vi "ff_retag_blocks.vi"(8 "error in (no error)":errorcluster) -> (0 "error out":errorcluster)   [LabVIEW 2016]
uses:
  Typedef/comm_variable_definition.ctl
  Typedef/Comm_mode_type_combo.ctl
  Typedef/Comm_mode_and_address_type.ctl
panel:
  in  "Comm variable definitions":T1[](array[typedef]) {"Cluster"."Mode" items=["None", "MODBUS", "HART", "Profibus DP", "Profibus PA", "Fieldbus", "DeviceNET"]}
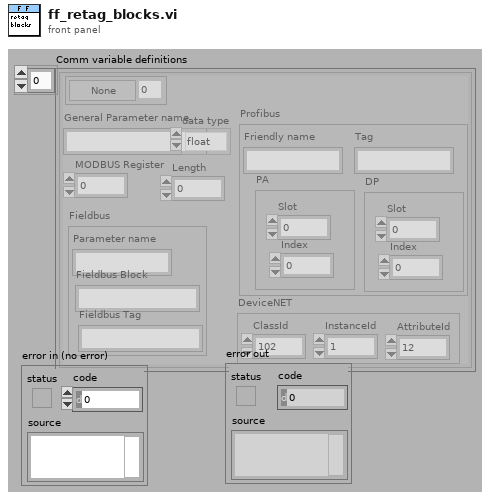
[diagram p1: front panel]
types:
  T1 = typedef "comm_variable_definition.ctl" = cluster{"General Parameter name":string, "MODBUS Register":i32, "Profibus":cluster{"Friendly name":string, "PA":cluster{"Slot":i32, "Index":i32}, "DP":cluster{"Slot":i32, "Index":i32}, "Tag":string}, "Fieldbus":cluster{"Parameter name":string, "Fieldbus Block":string, "Fieldbus Tag":string}, "data type":enum16{"float", "UINT", "UINT32", "STRING"}, "DeviceNET":cluster{"ClassId":u16, "InstanceId":u16, "AttributeId":u8}, "Cluster":T2, "Length":i32}
  T2 = typedef "Comm_mode_and_address_type.ctl" = cluster{"address":i32, "Mode":T3}
  T3 = typedef "Comm_mode_type_combo.ctl" = u16
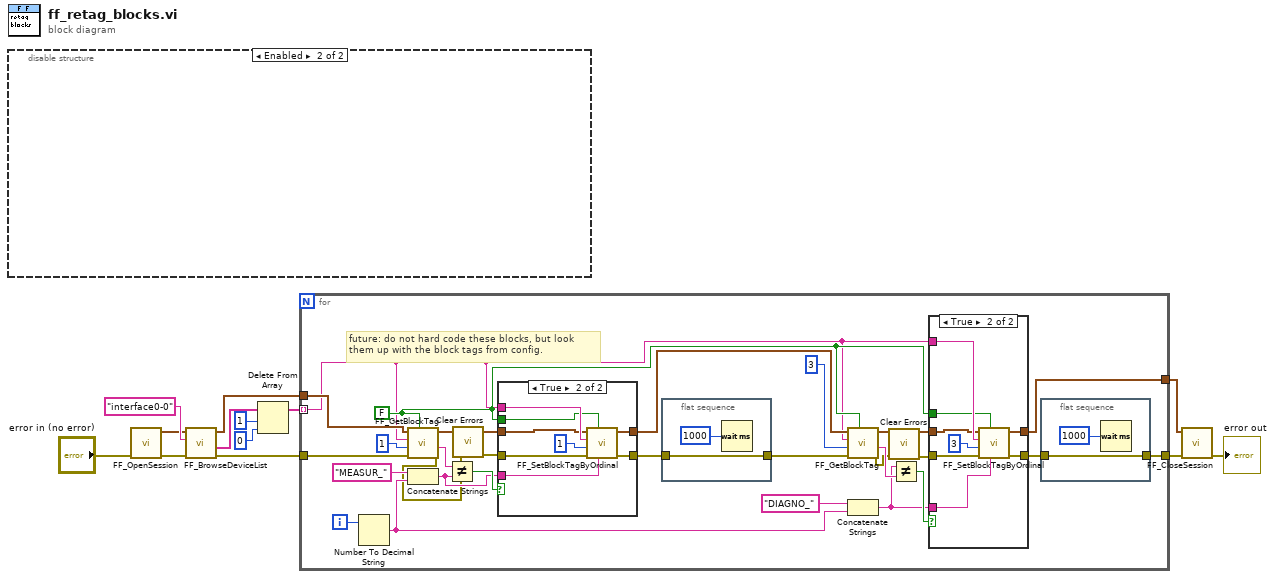
[diagram p0: block diagram]
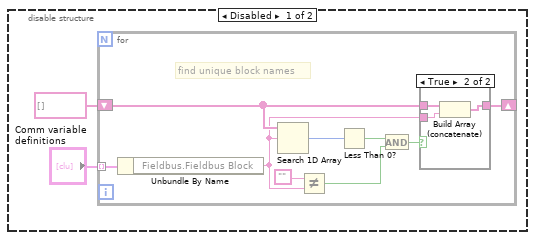
[diagram p2: hidden frame]
diagram:
  n1 = disable-structure shown="Enabled" {
    frame Disabled {
      n2 = for {
        tunnel: "Comm variable definitions" -> [w24] mode=indexing
        shift-right: [w21] -> _
        shift-left: string[] [] -> [w20]
        # "find unique block names"
        n3 = Unbundle By Name(w24) -> ("Fieldbus.Fieldbus Block"=w16:string)
        n4 = Search 1D Array(1D array=w20, element=w16) -> (index of element=w19:i32)  [unwired: 1 in]
        n5 = Not Equal?(x="", y=w16) -> (x != y?=w22:bool)
        n6 = Less Than 0?(x=w19) -> (x < 0?=w17:bool)
        n7 = And(x=w17, y=w22) -> (x .and. y?=w18:bool)
        n8 = case shown="True" w18 {
          tunnel: w16 -> [_ w28]
          tunnel: [w25 w27] -> w21
          tunnel: w20 -> [w25 w26]
          frame False {
          }
          frame True {
            n9 = Build Array (concatenate)(w26, w28) -> (w27:string[])
          }
        }
      }
    }
    frame Enabled {
    }
  }
  n10 = call "FF_OpenSession.vi"("error in (no error)"="error in (no error)") -> ("error out"=w9:errorcluster, "refnum out"=w8:cluster{"Handle1":u32, "Handle2":u32})  [unwired: 9 in]
  n11 = call "FF_BrowseDeviceList.vi"("error in (no error)"=w9, "link name"="interface0-0", "refnum in"=w8) -> ("error out"=w5:errorcluster, "deviceID list"=w13:string[], "refnum out"=w6:cluster{"Handle1":u32, "Handle2":u32})  [unwired: 4 in, 2 out]
  n12 = Delete From Array(array=w13, length=1, index=0) -> (array with subset deleted=w7:string[])  [unwired: 1 out]
  n13 = for {
    tunnel: w7 -> [w39] mode=indexing
    tunnel: [w33] -> w3
    tunnel: w6 -> [w52]
    tunnel: w5 -> [w47]
    tunnel: [w37] -> w4
    i -> [w55]
    w40 = FALSE ("Is pdTag")
    # "future: do not hard code these blocks, but look \nthem up with the block tags from config."
    n14 = Number To Decimal String(number=w55) -> (decimal integer string=w53:string)  [unwired: 1 in]
    n15 = call "FF_GetBlockTag.vi"("Is pdTag"=w40, "error in (no error)"=w47, "block ordinal"=u32 1, "pdTag/deviceID"=w39, "refnum in"=w52) -> ("error out"=w32:errorcluster, "block tag"=w50:string, "refnum out"=w48:cluster{"Handle1":u32, "Handle2":u32})  [unwired: 4 in]
    n16 = Concatenate Strings("MEASUR_" ("pdTag/deviceID"), w53) -> (w46:string)
    n17 = Not Equal?(x=w50, y=w46) -> (x != y?=w49:bool)
    n18 = call <vilib>:"Clear Errors.vi"("error in (no error)"=w32) -> ("error out"=w31:errorcluster)  [unwired: 5 in, 1 out]
    n19 = case shown="True" w49 {
      tunnel: w39 -> [_ w79]
      tunnel: w48 -> [w72 w78]
      tunnel: w31 -> [w71 w77]
      tunnel: [w71 w76] -> w36
      tunnel: w46 -> [_ w75]
      tunnel: w40 -> [_ w74]
      tunnel: [w72 w73] -> w45
      frame False {
      }
      frame True {
        n20 = call "FF_SetBlockTagByOrdinal.vi"("new block tag"=w75, "Is pdTag"=w74, "error in (no error)"=w77, "block ordinal"=u32 1, "pdTag/deviceID"=w79, "refnum in"=w78) -> ("error out"=w76:errorcluster, "refnum out"=w73:cluster{"Handle1":u32, "Handle2":u32})  [unwired: 4 in]
      }
    }
    n21 = flat-sequence {
      tunnel: w36 -> [w59]
      tunnel: [w59] -> w35
      frame #0 {
        n22 = Wait (ms)(milliseconds to wait=u32 1000) -> ()  [unwired: 1 out]
      }
    }
    n23 = call "FF_GetBlockTag.vi"("Is pdTag"=w40, "error in (no error)"=w35, "block ordinal"=u32 3, "pdTag/deviceID"=w39, "refnum in"=w45) -> ("error out"=w30:errorcluster, "block tag"=w43:string, "refnum out"=w41:cluster{"Handle1":u32, "Handle2":u32})  [unwired: 4 in]
    n24 = Concatenate Strings("DIAGNO_" ("pdTag/deviceID"), w53) -> (w38:string)
    n25 = call <vilib>:"Clear Errors.vi"("error in (no error)"=w30) -> ("error out"=w29:errorcluster)  [unwired: 5 in, 1 out]
    n26 = Not Equal?(x=w38, y=w43) -> (x != y?=w42:bool)
    n27 = case shown="True" w42 {
      tunnel: w39 -> [_ w69]
      tunnel: w41 -> [w62 w68]
      tunnel: w29 -> [w61 w67]
      tunnel: [w61 w66] -> w34
      tunnel: w38 -> [_ w65]
      tunnel: w40 -> [_ w64]
      tunnel: [w62 w63] -> w37
      frame False {
      }
      frame True {
        n28 = call "FF_SetBlockTagByOrdinal.vi"("new block tag"=w65, "Is pdTag"=w64, "error in (no error)"=w67, "block ordinal"=u32 3, "pdTag/deviceID"=w69, "refnum in"=w68) -> ("error out"=w66:errorcluster, "refnum out"=w63:cluster{"Handle1":u32, "Handle2":u32})  [unwired: 4 in]
      }
    }
    n29 = flat-sequence {
      tunnel: w34 -> [w57]
      tunnel: [w57] -> w33
      frame #0 {
        n30 = Wait (ms)(milliseconds to wait=u32 1000) -> ()  [unwired: 1 out]
      }
    }
  }
  n31 = call "FF_CloseSession.vi"("error in (no error)"=w3, "refnum in"=w4) -> ("error out"=→"error out":errorcluster)  [unwired: 9 in]
